vi "ProdaNG.Tree.TestStepParams.Add.vi"(4 "TS":T1, 5 "TS":i32, 6 "Mode":T3, 7 "TestStepsTree":refnum<vi>, 8 "error in (no error)":errorcluster, 9 "units":T5[](array[typedef]), 10 "testStepId":i32, 11 "dbHandleIn":i32) -> (0 "error out":errorcluster, 1 "#changes":i32, 2 "TestStepParams":T4[](array[typedef]) {"value" format="%#.3f"}, 3 "dbHandle":i32)   [LabVIEW 2016]
doc: "This function returns a product structure for a product, which is identified by a part and a serial number.\nImportant information: The field 'individual' was taken over from the field 'allgemein' of the legacy data directly. Because of this most products have the value 0 further on and only a few the value 1. \nParameter:\nhandle is an Integer, which is returned by the function Login() at the creation of a new connection.\nwabcoPartId is the Id of the part.\nserialNumber is the serial number of the product for the part above.\nproduct is a pointer on a product structure, which is filled if the returncode is 0. The structure must be defined in the calling program.\n\nReturncodes:\n0 No error\n< 0 ORACLE Error code\n6 (ERROR_INVALID_HANDLE) in case of an invalid handle\n1403 Record does not exist"
uses:
  Controls/ProdaNG.UnitSimple.ctl
  Controls/ProdaNG.TestStepParam.ctl
  ProdaNG.Tree.TestViewMode.ctl
  ProdaNG.File.Step.ctl
  ProdaNG.Tree.Fglb.Value.ctl
  ProdaNG.Tree.Fglb.Data.ctl
  ProdaNG.Tree.Fglb.Element.ctl
  ProdaNG.Tree.Fglb.Action.ctl
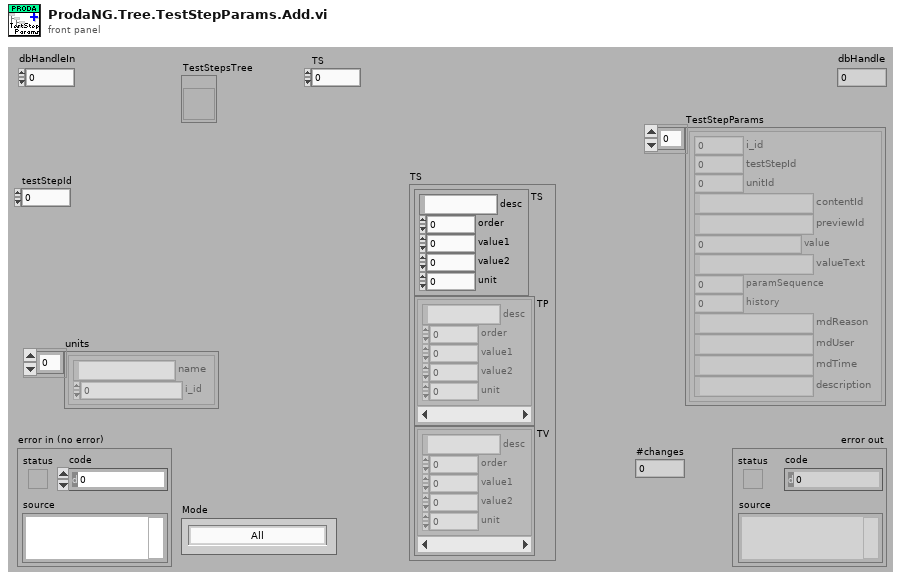
[diagram p1: front panel]
types:
  T1 = typedef "ProdaNG.File.Step.ctl" = cluster{"TS":T2, "TP":T2[], "TV":T2[]}
  T2 = typedef "ProdaNG.Tree.Fglb.Value.ctl" = cluster{"desc":string, "order":i32, "value1":dbl, "value2":dbl, "unit":i32}
  T3 = typedef "ProdaNG.Tree.TestViewMode.ctl" = enum16{"All", "Released", "Unreleased"}
  T4 = typedef "ProdaNG.TestStepParam.ctl" = cluster{"i_id":i32, "testStepId":i32, "unitId":i32, "contentId":string, "previewId":string, "value":dbl, "valueText":string, "paramSequence":i32, "history":i32, "mdReason":string, "mdUser":string, "mdTime":string, "description":string}
  T5 = typedef "ProdaNG.UnitSimple.ctl" = cluster{"name":string, "i_id":i32}
  T6 = typedef "ProdaNG.Tree.Fglb.Action.ctl" = enum16{"init", "add", "get by row", "get by tag", "get by idx"}
  T7 = typedef "ProdaNG.Tree.Fglb.Element.ctl" = enum16{"-", "PP", "TS", "TP", "TV"}
  T8 = typedef "ProdaNG.Tree.Fglb.Data.ctl" = cluster{"tag":string, "row":i32, "element":T7, "idx1":i32, "idx2":i32, "file":bool}
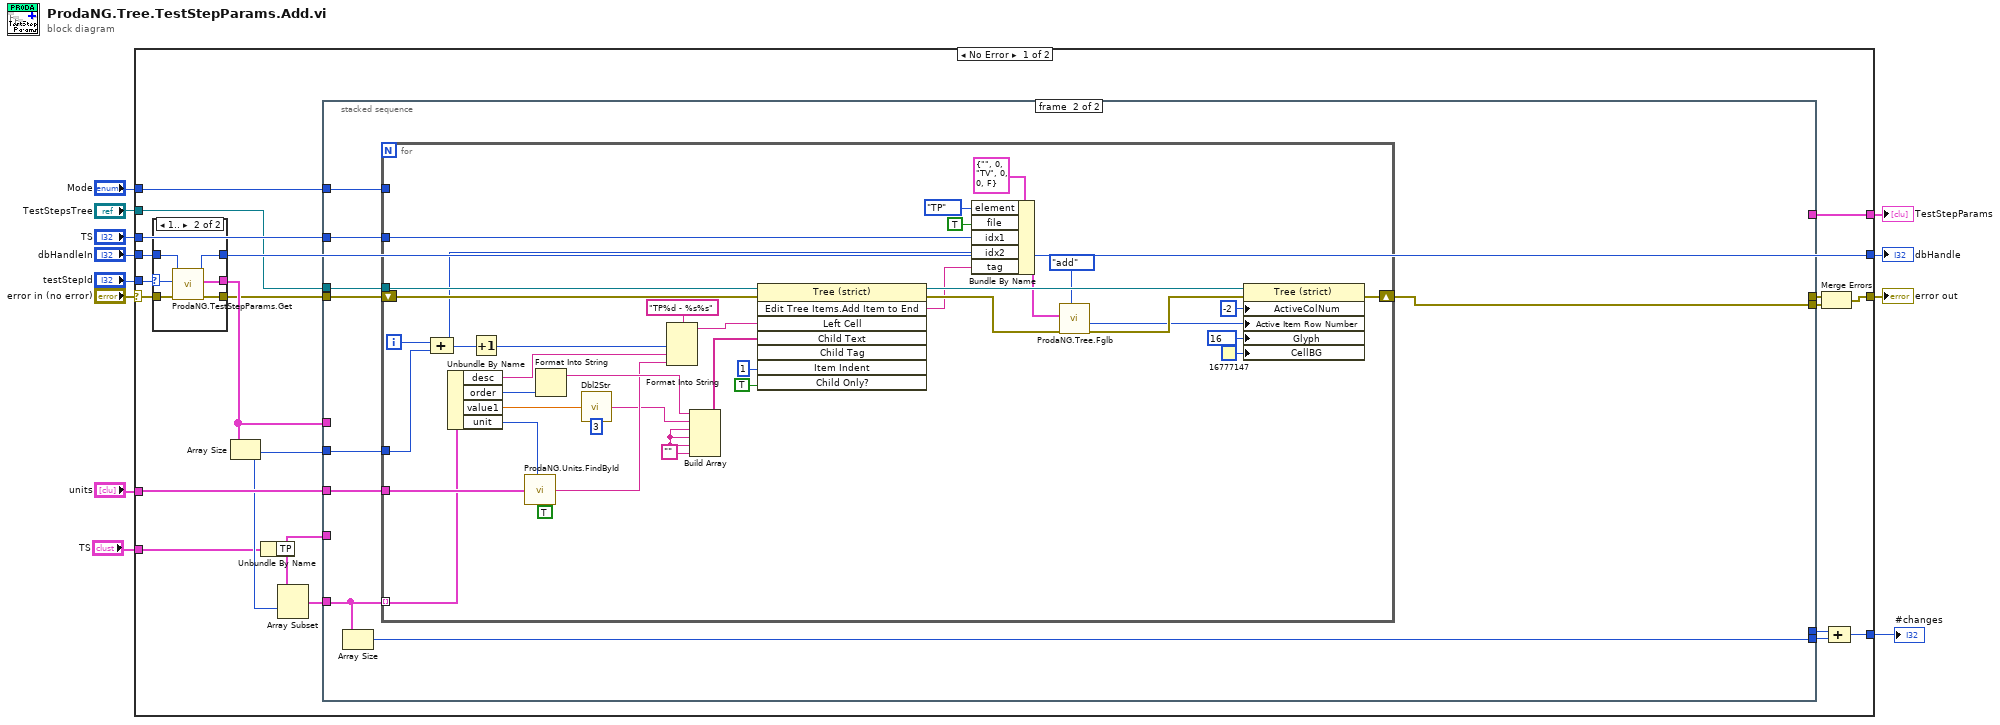
[diagram p0: block diagram]
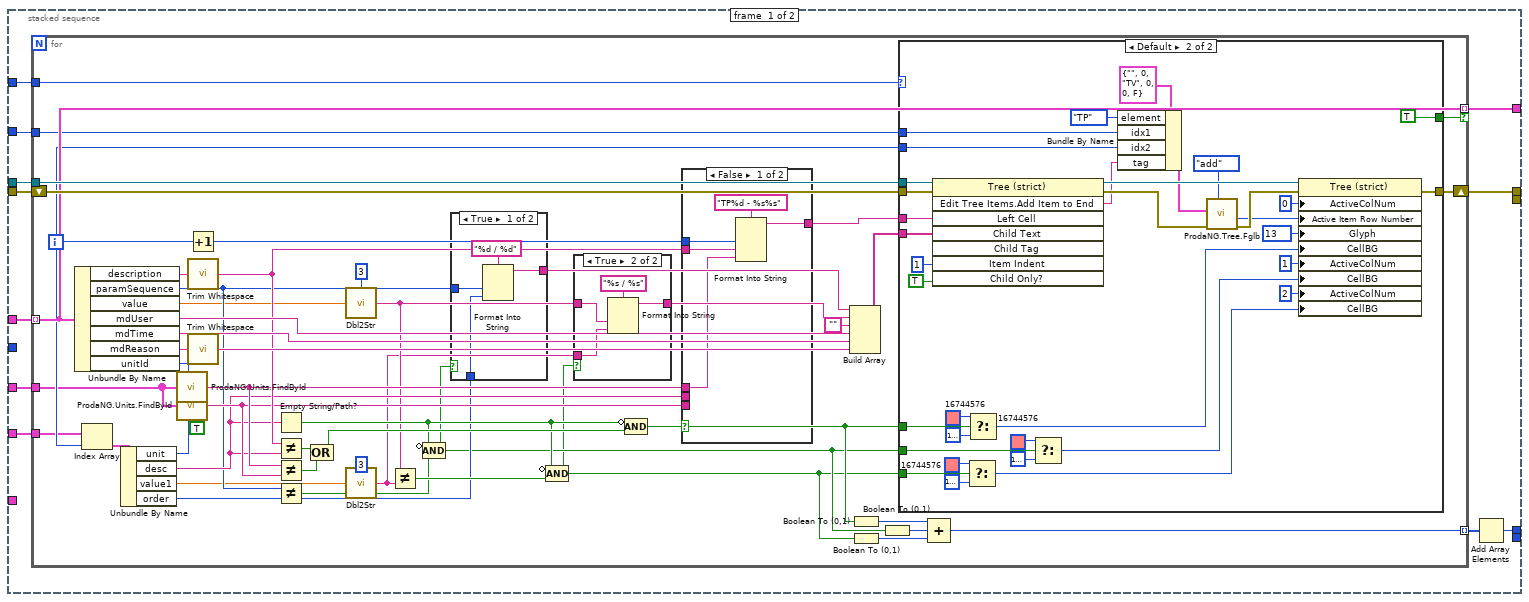
[diagram p3: hidden frame]
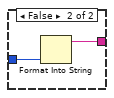
[diagram p4: hidden frame]
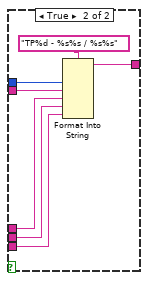
[diagram p6: hidden frame]
diagram:
  n1 = case shown="No Error" "error in (no error)" {
    selector: "error in (no error)" -> [w33 w210]
    tunnel: [w20 w210] -> w9
    tunnel: "dbHandleIn" -> [w32 w209]
    tunnel: [w31 w209] -> w8
    tunnel: "testStepId" -> [w16 _]
    tunnel: "units" -> [w28 _]
    tunnel: "TestStepsTree" -> [w23 _]
    tunnel: [w18 _] -> w5
    tunnel: "TS" -> [w26 _]
    tunnel: "Mode" -> [w25 _]
    tunnel: "TS" -> [w17 _]
    tunnel: [w14 _] -> w1
    frame No Error {
      n2 = case shown="1.." w16 {
        selector: w16 -> [_ w36]
        tunnel: w33 -> [w34 w41]
        tunnel: w32 -> [w35 w40]
        tunnel: [w35 w39] -> w31
        tunnel: [_ w38] -> w27
        tunnel: [w34 w37] -> w24
        frame Default {
        }
        frame 1.. {
          n3 = call "ProdaNG.TestStepParams.Get.vi"("error in (no error)"=w41, "testStepId"=w36, "dbHandleIn"=w40) -> ("error out"=w37:errorcluster, "TestStepParams"=w38:T4[], "dbHandle"=w39:i32)  [unwired: 6 in]
        }
      }
      n4 = Array Size(array=w27) -> (size(s)=w21:i32)
      n5 = Unbundle By Name(w17) -> ("TP"=w22:T2[])
      n6 = Array Subset(array=w22, index=w21) -> (w30:T2[])  [unwired: 1 in]
      n7 = stacked-sequence {
        tunnel: [w52 _] -> w29
        tunnel: w24 -> [w51 w170]
        tunnel: w23 -> [w50 w169]
        tunnel: w25 -> [w49 w168]
        tunnel: [w48 _] -> w18
        tunnel: w28 -> [w47 w167]
        tunnel: w22 -> [w46 _]
        tunnel: w27 -> [w45 _]
        tunnel: w30 -> [_ w163]
        tunnel: w21 -> [_ w164]
        tunnel: w26 -> [w44 w166]
        tunnel: [_ w165] -> w19
        tunnel: [w42 _] -> w15
        tunnel: [_ w162] -> w13
        frame #0 {
          n8 = for {
            shift-right: [w94] -> w52
            shift-left: w51 -> [w102]
            tunnel: w45 -> [w89] mode=indexing
            tunnel: w50 -> [w98]
            tunnel: w49 -> [w91]
            tunnel: [w89] -> w48 mode=indexing if=w88
            tunnel: w47 -> [w78]
            tunnel: w46 -> [w85]
            tunnel: w44 -> [w67]
            tunnel: [w54] -> w43 mode=indexing
            i -> [w86]
            w53 = TRUE ("add quotas (F)")
            n9 = Unbundle By Name(w89) -> ("description"=w87:string, "paramSequence"=w71:i32, "value"=w64:dbl, "mdUser"=w100:string, "mdTime"=w101:string, "mdReason"=w97:string, "unitId"=w80:i32)
            n10 = Index Array(array=w85, index=w86) -> (element=w84:T2)
            n11 = Unbundle By Name(w84) -> ("unit"=w79:i32, "desc"=w74:string, "value1"=w63:dbl, "order"=w69:i32)
            n12 = call "ProdaNG.Units.FindById.vi"("units"=w78, "unit id"=w80, "add brackets (F)"=w53) -> ("unit str"=w77:string)
            n13 = call "ProdaNG.Units.FindById.vi"("units"=w78, "unit id"=w79, "add brackets (F)"=w53) -> ("unit str"=w76:string)
            n14 = Increment(x=w86) -> (x+1=w95:i32)
            n15 = call <vilib>:"Trim Whitespace.vi"("string"=w87) -> ("trimmed string"=w83:string)  [unwired: 1 in]
            n16 = call <vilib>:"Trim Whitespace.vi"("string"=w97) -> ("trimmed string"=w93:string)  [unwired: 1 in]
            n17 = Empty String/Path?(string/path=w74) -> (empty?=w72:bool)
            n18 = Not Equal?(x=w83, y=w74) -> (x != y?=w82:bool)
            n19 = Not Equal?(x=w77, y=w76) -> (x != y?=w81:bool)
            n20 = Not Equal?(x=w71, y=w69) -> (x != y?=w70:bool)
            n21 = Compound Arithmetic op=OR(w82, w81) -> (w75:bool)
            n22 = call "Dbl2Str.vi"("Numeric"=w64, "precision (6)"=i16 3) -> ("string"=w66:string)
            n23 = call "Dbl2Str.vi"("Numeric"=w63, "precision (6)"=i16 3) -> ("string"=w62:string)
            n24 = Not Equal?(x=w66, y=w62) -> (x != y?=w73:bool)
            n25 = Compound Arithmetic op=AND(invert w72, w70) -> (w56:bool)
            n26 = case shown="True" w56 {
              tunnel: w71 -> [w106 w108]
              tunnel: [w105 w107] -> w92
              tunnel: w69 -> [w103 _]
              frame True {
                n27 = Format Into String(format string="%d / %d", w106, w103) -> (resulting string=w105:string)  [unwired: 2 in, 1 out]
              }
              frame False {
                n28 = Format Into String(w108) -> (resulting string=w107:string)  [unwired: 3 in, 1 out]
              }
            }
            n29 = Compound Arithmetic op=AND(invert w72, w73) -> (w55:bool)
            n30 = case shown="True" w55 {
              tunnel: [w109 w112] -> w96
              tunnel: w66 -> [w109 w111]
              tunnel: w62 -> [_ w110]
              frame False {
              }
              frame True {
                n31 = Format Into String(format string="%s / %s", w111, w110) -> (resulting string=w112:string)  [unwired: 2 in, 1 out]
              }
            }
            n32 = Compound Arithmetic op=AND(invert w72, w75) -> (w57:bool)
            n33 = case shown="False" w57 {
              tunnel: w77 -> [w114 w121]
              tunnel: w95 -> [w117 w124]
              tunnel: w83 -> [w116 w123]
              tunnel: [w115 w122] -> w90
              tunnel: w74 -> [_ w120]
              tunnel: w76 -> [_ w119]
              frame False {
                n34 = Format Into String(format string="TP%d - %s%s", w117, w116, w114) -> (resulting string=w115:string)  [unwired: 2 in, 1 out]
              }
              frame True {
                n35 = Format Into String(format string="TP%d - %s%s / %s%s", w124, w123, w121, w120, w119) -> (resulting string=w122:string)  [unwired: 2 in, 1 out]
              }
            }
            n36 = Build Array(w92, w96, "", w100, w101, w93) -> (w99:string[])
            n37 = Boolean To (0,1)(Boolean=w57) -> (0, 1=w60:i16)
            n38 = Boolean To (0,1)(Boolean=w55) -> (0, 1=w58:i16)
            n39 = Boolean To (0,1)(Boolean=w56) -> (0, 1=w59:i16)
            n40 = case shown="Default" w91 {
              tunnel: w102 -> [w126 w159]
              tunnel: w90 -> [_ w158]
              tunnel: w99 -> [_ w157]
              tunnel: w98 -> [_ w156]
              tunnel: [w126 w150] -> w94
              tunnel: w86 -> [_ w147]
              tunnel: [_ TRUE] -> w88
              tunnel: w57 -> [_ w141]
              tunnel: w56 -> [_ w135]
              tunnel: w55 -> [_ w130]
              tunnel: w67 -> [_ w127]
              frame "Unreleased" {
              }
              frame Default {
                n41 = invoke on="Invoke Node" class="Tree (strict)" method="Edit Tree Items.Add Item to End"(reference=w156, error in=w159, "Left Cell"=w158, "Child Text"=w157, "Item Indent"=1 ("New Item Indentation"), "Child Only?"=TRUE) -> (reference out=w152:refnum<vi>, error out=w145:errorcluster, "Edit Tree Items:Add Item to End"=w142:string)  [unwired: 2 in, 5 out]
                n42 = Select(t=u32 16744576, s=w130, f=u32 16777225) -> (s? t:f=w129:u32)
                n43 = Select(t=u32 16744576, s=w141, f=u32 16777225) -> (s? t:f=w128:u32)
                n44 = Select(t=u32 16744576, s=w135, f=u32 16777225) -> (s? t:f=w134:u32)
                n45 = Bundle By Name(cluster=T8 {"tag"="", "row"=0, "element"=enum."TV", "idx1"=0, "idx2"=0, "file"=FALSE} ("entry in"), "element"=ProdaNG.Tree.Fglb.Element."TP", "idx1"=w127, "idx2"=w147, "tag"=w142) -> (w146:T8)
                n46 = call "ProdaNG.Tree.Fglb.vi"("Action (add)"=ProdaNG.Tree.Fglb.Action."add", "error in"=w145, "entry in"=w146) -> ("error out"=w153:errorcluster, "active row"=w151:i32)  [unwired: 6 in, 1 out]
                n47 = property class="Tree (strict)"(reference=w152, error in=w153, "ActiveColNum"=0 ("Active Cell:Active Column Number"), "Active Item Row Number"=w151, "Glyph"=13, "CellBG"=w128, "ActiveColNum"=1 ("Active Cell:Active Column Number"), "CellBG"=w134, "ActiveColNum"=2 ("Active Cell:Active Column Number"), "CellBG"=w129) -> (error out=w150:errorcluster)  [unwired: 1 out]
              }
            }
            n48 = Compound Arithmetic op=ADD(w60, w59, w58) -> (w54:i16)
          }
          n49 = Add Array Elements(numeric array=w43) -> (sum=w42:i16)
        }
        frame #1 {
          n50 = Array Size(array=w163) -> (size(s)=w162:i32)
          n51 = for {
            shift-right: [w204] -> w165
            shift-left: w170 -> [w208]
            tunnel: w169 -> [w206]
            tunnel: w168 -> [_]
            tunnel: w167 -> [w198]
            tunnel: w163 -> [w190] mode=indexing
            tunnel: w164 -> [w187]
            tunnel: w166 -> [w175]
            i -> [w200]
            w176 = ""
            n52 = Compound Arithmetic op=ADD(w200, w187) -> (w179:i32)
            n53 = Unbundle By Name(w190) -> ("desc"=w201:string, "order"=w196:i32, "value1"=w173:dbl, "unit"=w199:i32)
            n54 = Increment(x=w179) -> (x+1=w205:i32)
            n55 = call "ProdaNG.Units.FindById.vi"("units"=w198, "unit id"=w199, "add brackets (F)"=TRUE ("add quotas (F)")) -> ("unit str"=w197:string)
            n56 = Format Into String(w196) -> (resulting string=w203:string)  [unwired: 3 in, 1 out]
            n57 = call "Dbl2Str.vi"("Numeric"=w173, "precision (6)"=i16 3) -> ("string"=w172:string)
            n58 = Format Into String(format string="TP%d - %s%s", w205, w201, w197) -> (resulting string=w202:string)  [unwired: 2 in, 1 out]
            n59 = Build Array(w203, w172, w176, w176, w176, w176) -> (w207:string[])
            n60 = invoke on="Invoke Node" class="Tree (strict)" method="Edit Tree Items.Add Item to End"(reference=w206, error in=w208, "Left Cell"=w202, "Child Text"=w207, "Item Indent"=1 ("New Item Indentation"), "Child Only?"=TRUE) -> (reference out=w191:refnum<vi>, error out=w183:errorcluster, "Edit Tree Items:Add Item to End"=w180:string)  [unwired: 2 in, 5 out]
            n61 = Bundle By Name(cluster=T8 {"tag"="", "row"=0, "element"=enum."TV", "idx1"=0, "idx2"=0, "file"=FALSE} ("entry in"), "element"=ProdaNG.Tree.Fglb.Element."TP", "file"=TRUE, "idx1"=w175, "idx2"=w179, "tag"=w180) -> (w181:T8)
            n62 = call "ProdaNG.Tree.Fglb.vi"("Action (add)"=ProdaNG.Tree.Fglb.Action."add", "error in"=w183, "entry in"=w181) -> ("error out"=w182:errorcluster, "active row"=w177:i32)  [unwired: 6 in, 1 out]
            n63 = property class="Tree (strict)"(reference=w191, error in=w182, "ActiveColNum"=-2 ("Active Cell:Active Column Number"), "Active Item Row Number"=w177, "Glyph"=16, "CellBG"=u32 16777147) -> (error out=w204:errorcluster)  [unwired: 1 out]
          }
        }
      }
      n64 = Merge Errors(w29, w19) -> (w20:errorcluster)
      n65 = Compound Arithmetic op=ADD(w15, w13) -> (w14:i32)
    }
    frame Error {
    }
  }
  "error out" <- w9
  "dbHandle" <- w8
  "TestStepParams" <- w5
  "#changes" <- w1
